vi "(SubVI)_ UpdateStimGalvoCluster.vi"(1 "X and Y Values":dbl[](array[numeric]), 2 "Galvo Template":T1) -> (0 "Stim Galvo Cluster":T1)   [LabVIEW 2019]
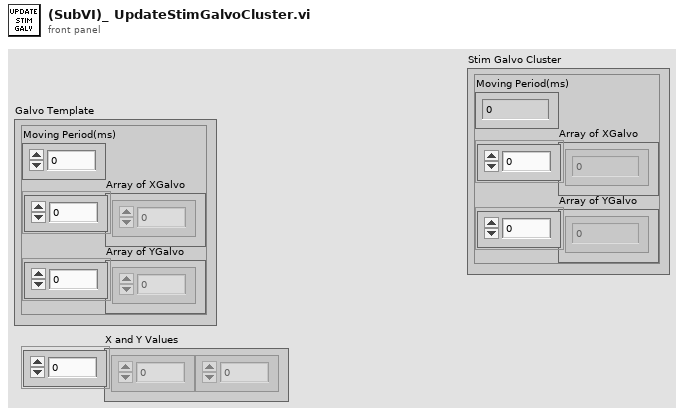
[diagram p1: front panel]
types:
  T1 = cluster{"Moving Period(ms)":dbl, "Array of XGalvo":dbl[], "Array of YGalvo":dbl[]}
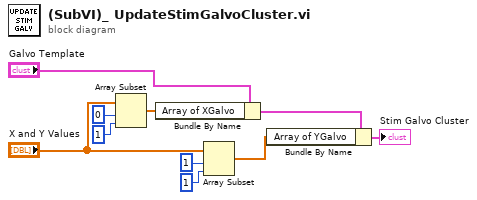
[diagram p0: block diagram]
diagram:
  n1 = Array Subset(array="X and Y Values", index=0, length=1) -> (w8:dbl[])
  n2 = Bundle By Name(cluster="Galvo Template", "Array of XGalvo"=w8) -> (w2:T1)
  n3 = Array Subset(array="X and Y Values", index=1, length=1) -> (w3:dbl[])
  n4 = Bundle By Name(cluster=w2, "Array of YGalvo"=w3) -> (→"Stim Galvo Cluster":T1)
